vi "DN4_AI_ReadScaledData.vi"(4 "error in (no error)":errorcluster, 5 "count":i32, 7 "Task ID":u32) -> (0 "error out":errorcluster, 1 "data":dbl[](array[numeric]), 2 "start time":dbl, 3 "Task ID":u32)   [LabVIEW 2009]
uses:
  Windows/System32/AdvLvDaq.dll
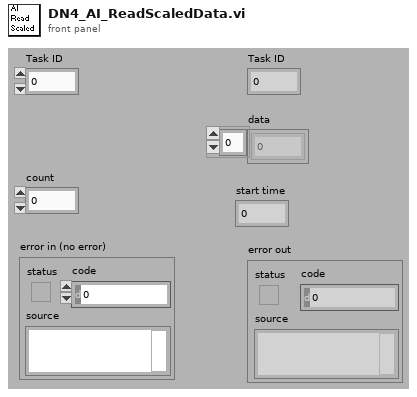
[diagram p1: front panel]
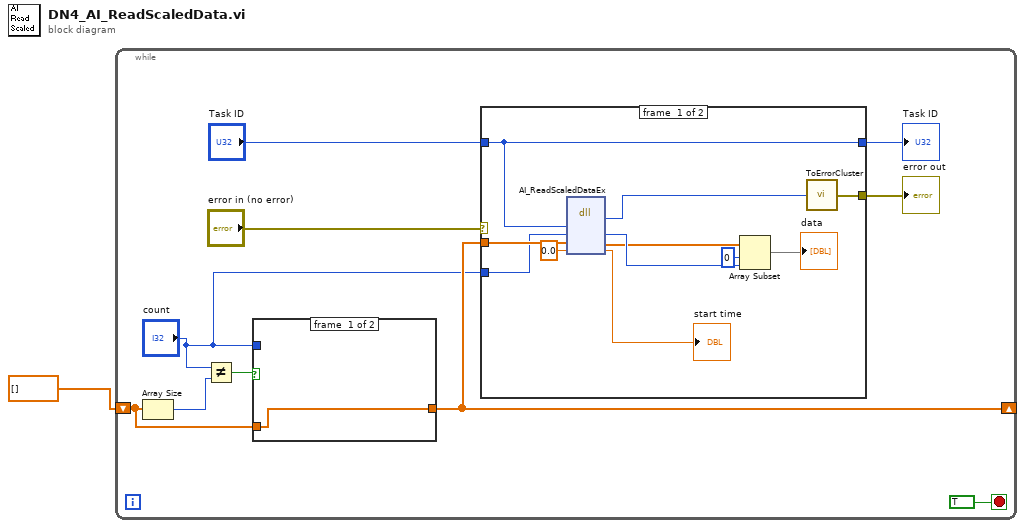
[diagram p0: block diagram]
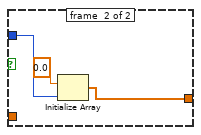
[diagram p2: hidden frame]
diagram:
  n1 = while {
    shift-right: [w3] -> _
    shift-left: dbl[] [] -> [w4]
    stop <- TRUE stop-if-true
    n2 = Array Size(array=w4) -> (size(s)=w6:i32)
    n3 = Not Equal?(x="count", y=w6) -> (x != y?=w5:bool)
    n4 = case shown="True" w5 {
      tunnel: "count" -> [_ w15]
      tunnel: [w12 w13] -> w3
      tunnel: w4 -> [w12 _]
      frame #0 {
      }
      frame #1 {
        n5 = Initialize Array(0.0 ("element"), w15) -> (w13:dbl[])
      }
    }
    n6 = case shown="No Error" "error in (no error)" {
      selector: "error in (no error)" -> [_ w28]
      tunnel: "Task ID" -> [w24 w27]
      tunnel: [w25 w28] -> w9
      tunnel: [w24 w27] -> w8
      tunnel: w3 -> [w19 _]
      tunnel: "count" -> [w18 _]
      frame #0 {
        n7 = dll-call lib="C:/Windows/System32/AdvLvDaq.dll" fn="AI_ReadScaledDataEx"("taskId"=w24, "count"=w18, "data"=w19, "startTime"=0.0) -> ("return type"=w26:i32, "count"=w22:i32, "data"=w21:dbl[], "startTime"=→"start time":dbl)  [unwired: 4 in, 2 out]
        n8 = Array Subset(array=w21, index=0, length=w22) -> (→"data":dbl[])
        n9 = call <userlib>:"ToErrorCluster.vi"("error code"=w26) -> ("error out"=w25:errorcluster)
      }
      frame #1 {
      }
    }
    "error out" <- w9
    "Task ID" <- w8
  }
